vi "Test Command RPORT Response.vi"(8 "error in (no error)":errorcluster, 11 "TestCase in":refnum<class "Test ADC Command.lvclass">) -> (0 "error out":errorcluster, 3 "TestCase out":refnum<class "Test ADC Command.lvclass">)   [LabVIEW 2019, in "Test ADC Command.lvclass"]
uses:
  Test ADC Command.lvclass
  SIMULATED/SIMULATED.lvclass
  <vilib>/addons/_JKI Toolkits/VI Tester/TestCase.llb/TestCase.lvclass
  Serial Devices.lvclass
  C:/Program Files (x86)/National Instruments/LabVIEW 2019/vi.lib/addons/_JKI Toolkits/VI Tester/TestCase.llb/TestCase.lvclass
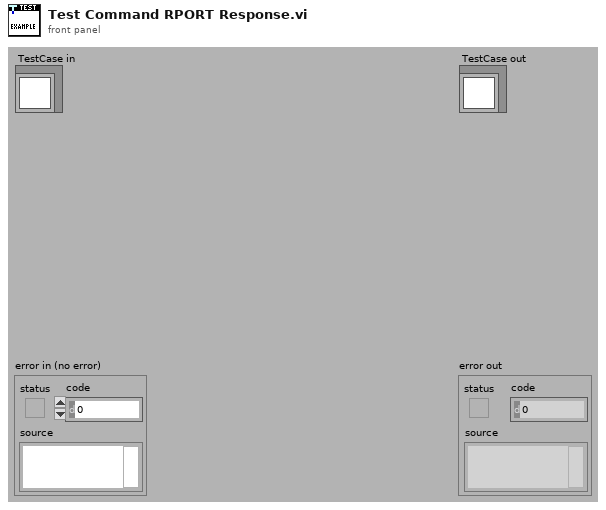
[diagram p1: front panel]
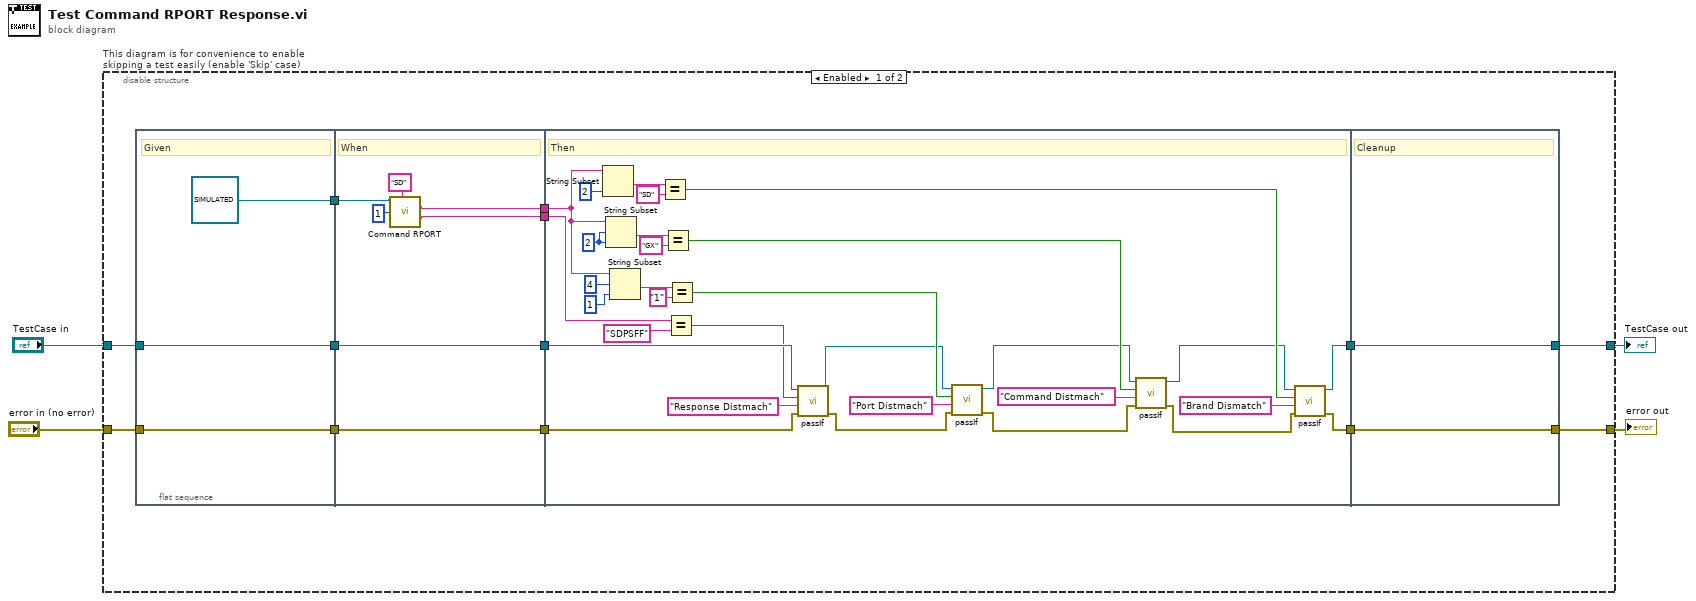
[diagram p0: block diagram]
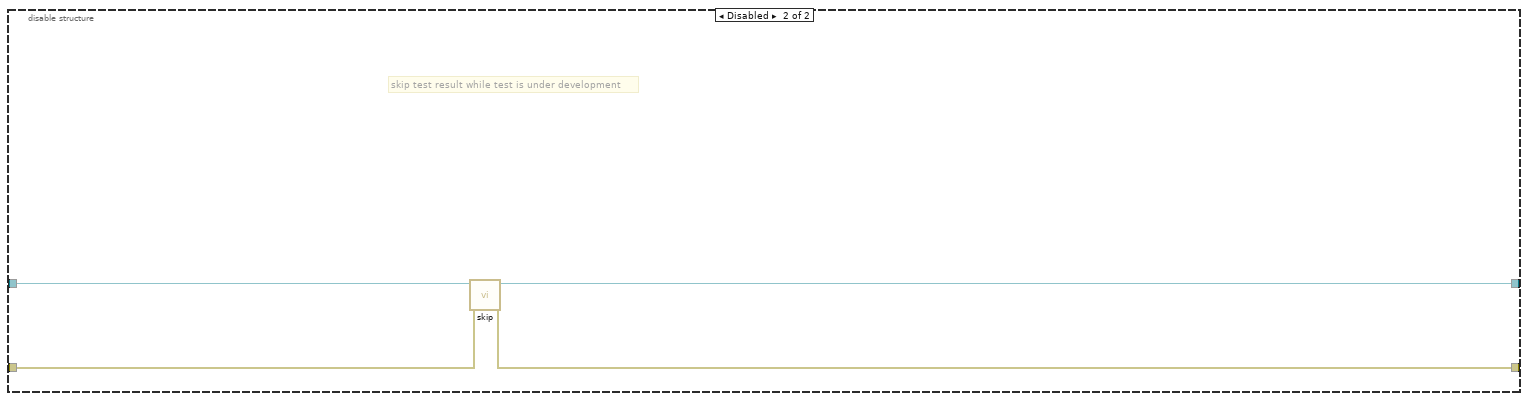
[diagram p2: hidden frame]
diagram:
  n1 = disable-structure "This diagram is for convenience to enable skipping a test easily (enable 'Skip' case)" shown="Enabled" {
    disable-tunnel: "TestCase in" -> [w16 w64]
    disable-tunnel: [w9 w62] -> w3
    disable-tunnel: [w8 w63] -> w4
    disable-tunnel: "error in (no error)" -> [w13 w61]
    frame Enabled {
      n2 = flat-sequence {
        tunnel: [w20] -> w17
        tunnel: w16 -> [w20]
        tunnel: [w19] -> w14
        tunnel: w13 -> [w19]
        tunnel: [refnum<class "SIMULATED.lvclass"> refnum ("SIMULATED.lvclass")] -> w7
        tunnel: w17 -> [w26]
        tunnel: [w26] -> w15
        tunnel: w14 -> [w27]
        tunnel: [w27] -> w12
        tunnel: w7 -> [w25]
        tunnel: [w23] -> w6
        tunnel: [w22] -> w5
        tunnel: w15 -> [w32]
        tunnel: w12 -> [w29]
        tunnel: [w53] -> w11
        tunnel: [w54] -> w10
        tunnel: w6 -> [w36]
        tunnel: w5 -> [w35]
        tunnel: [w60] -> w9
        tunnel: w11 -> [w60]
        tunnel: [w59] -> w8
        tunnel: w10 -> [w59]
        frame #0 {
          # "Given"
        }
        frame #1 {
          # "When"
          n3 = call "Command RPORT.vi"("Serial Devices in"=w25, "Device"="SD", "Port"=u8 1 ("Chanel")) -> ("Command"=w23:string, "Expected"=w22:string)  [unwired: 9 in, 2 out]
        }
        frame #2 {
          w49 = 2 ("offset (0)")
          # "Then"
          n4 = String Subset(string=w36, length (rest)=2 ("offset (0)")) -> (substring=w57:string)  [unwired: 1 in]
          n5 = String Subset(string=w36, offset (0)=w49, length (rest)=w49) -> (substring=w50:string)
          n6 = String Subset(string=w36, offset (0)=4, length (rest)=1 ("length (rest)")) -> (substring=w40:string)
          n7 = Equal?(x=w57, y="SD") -> (x = y?=w55:bool)
          n8 = Equal?(x=w50, y="GX") -> (x = y?=w47:bool)
          n9 = Equal?(x=w35, y="SDPSFF") -> (x = y?=w28:bool)
          n10 = Equal?(x=w40, y="1") -> (x = y?=w37:bool)
          n11 = call-dynamic "passIf.vi"("error in (no error)"=w29, "message (\"\")"="Response Distmach" ("message (\"\")"), "pass"=w28, "TestCase in"=w32) -> ("error out"=w30:errorcluster, "TestCase out"=w31:refnum<class "Test ADC Command.lvclass">)  [unwired: 6 in]
          n12 = call-dynamic "passIf.vi"("error in (no error)"=w30, "message (\"\")"="Port Distmach" ("message (\"\")"), "pass"=w37, "TestCase in"=w31) -> ("error out"=w43:errorcluster, "TestCase out"=w45:refnum<class "Test ADC Command.lvclass">)  [unwired: 6 in]
          n13 = call-dynamic "passIf.vi"("error in (no error)"=w43, "message (\"\")"="Command Distmach" ("message (\"\")"), "pass"=w47, "TestCase in"=w45) -> ("error out"=w42:errorcluster, "TestCase out"=w48:refnum<class "Test ADC Command.lvclass">)  [unwired: 6 in]
          n14 = call-dynamic "passIf.vi"("error in (no error)"=w42, "message (\"\")"="Brand Dismatch" ("message (\"\")"), "pass"=w55, "TestCase in"=w48) -> ("error out"=w54:errorcluster, "TestCase out"=w53:refnum<class "Test ADC Command.lvclass">)  [unwired: 6 in]
        }
        frame #3 {
          # "Cleanup"
        }
      }
    }
    frame Disabled {
      # "skip test result while test is under development"
      n15 = call <vilib>:"skip.vi"("error in (no error)"=w61, "TestCase in"=w64) -> ("error out"=w63:errorcluster, "TestCase out"=w62:refnum<class "Test ADC Command.lvclass">)  [unwired: 8 in]
    }
  }
  "error out" <- w4
  "TestCase out" <- w3
